vi "mod_Error Codes.vi"(1 "error condition enum":T1) -> (0 "error out":errorcluster)   [LabVIEW 2020, in "niAMT.lvlib"]
doc: "This VI sets the error code and status appropriately for the selected error condition."
uses:
  <vilib>/addons/Modulation/niAMT.lvlib
  <vilib>/addons/Modulation/Analog/controls/mod_Error Conditions.ctl
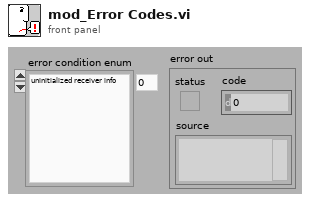
[diagram p1: front panel]
types:
  T1 = typedef "niAMT.lvlib/mod_Error Conditions.ctl" = enum16{"uninitialized receiver info", "invalid tuner task id", "invalid niScope handle", "unsupported receiver", "receiver mismatch", "null variant in IQ ViRef table", "RF attenuation value coerced", "FM deviation inconsistent with sample rate", "passband inconsistent with carrier frequency", "create mutex error (before DLL load attempt)", "DLL load error", "function not found in DLL", "handle dispose error", "invalid VI name from refnum", "cannot get attribute from new instance", "invalid session handle", "internal modulation toolkit error", "error loading dynamic VI for receiver", "requested downconversion inconsistent with sample rate", "failed to design downconversion filter", "invalid modulation index", "invalid pilot tone frequency", "invalid Hilbert filter taps", "invalid VSB filter taps ", "invalid VSB filter design (Nyquist)", "invalid VSB filter design (upper<=lower)", "invalid pilot search parameter(s)", "invalid dT", "invalid downconversion filter bandwidth", "modulation index exceeds one"}
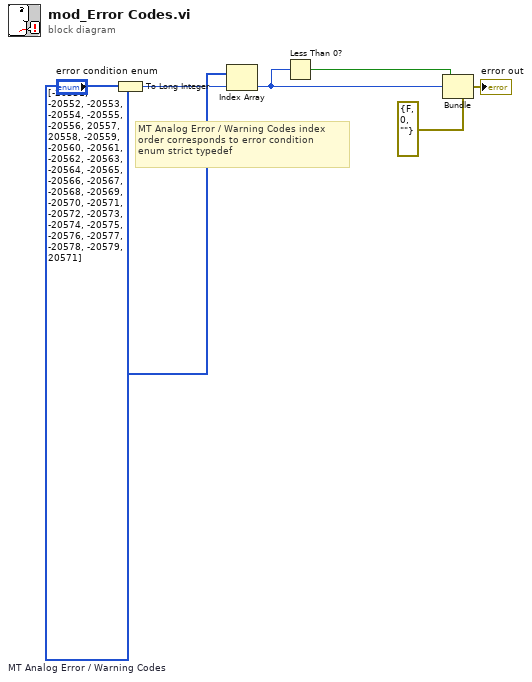
[diagram p0: block diagram]
diagram:
  w4 = i32[] [-20551, -20552, -20553, -20554, -20555, -20556, 20557, 20558, -20559, -20560, -20561, -20562, -20563, -20564, -20565, -20566, -20567, -20568, -20569, -20570, -20571, -20572, -20573, -20574, -20575, -20576, -20577, -20578, -20579, 20571]  # MT Analog Error / Warning Codes
  # "MT Analog Error / Warning Codes index\norder corresponds to error condition\nenum strict typedef"
  n1 = To Long Integer(number="error condition enum") -> (32bit integer=w3:i32)
  n2 = Index Array(array=w4, index=w3) -> (element=w1:i32)
  n3 = Less Than 0?(x=w1) -> (x < 0?=w2:bool)
  n4 = Bundle(cluster=errorcluster {"status"=FALSE, "code"=0, "source"=""} ("error out"), "status"=w2, "code"=w1) -> (→"error out":errorcluster)  [unwired: 1 out]
